vi "bpm.vi"() -> ()   [LabVIEW 2009, in "features.lvlib"]
doc: "The bpm vi uses the source rio to control the bpms on the high voltage deck. It can only work if the source rio is in the same project as this vi."
uses:
  Features/features/New Folder/features.lvlib
panel:
  out "error out":errorcluster
  in  "stop":bool
  in  "Source 2 X10":bool
  in  "Source 2 BPM":bool
  in  "Source 1 X 10":bool
  in  "Source 1 BPM":bool
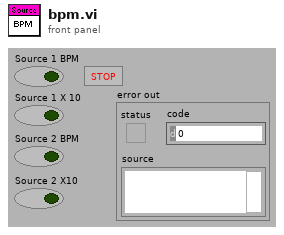
[diagram p1: front panel]
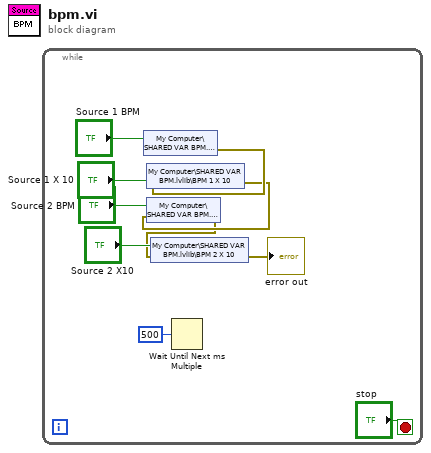
[diagram p0: block diagram]
diagram:
  n1 = while {
    stop <- "stop" stop-if-true
    n2 = shared-variable "My Computer\\SHARED VAR BPM.lvlib\\BPM 1"("Source 1 BPM") -> (error out=w4:errorcluster)  [unwired: 1 out]
    n3 = shared-variable "My Computer\\SHARED VAR BPM.lvlib\\BPM 1 X 10"("Source 1 X 10", error in=w4) -> (error out=w3:errorcluster)
    n4 = shared-variable "My Computer\\SHARED VAR BPM.lvlib\\BPM 2"("Source 2 BPM", error in=w3) -> (error out=w2:errorcluster)
    n5 = shared-variable "My Computer\\SHARED VAR BPM.lvlib\\BPM 2 X 10"("Source 2 X10", error in=w2) -> (error out=→"error out":errorcluster)
    n6 = Wait Until Next ms Multiple(millisecond multiple=u32 500) -> ()  [unwired: 1 out]
  }
